vi "To String.vi"(8 "error in (no error)":errorcluster, 11 "Variant in":refnum<class "Variant.lvclass">) -> (0 "error out":errorcluster, 2 "String":string)   [LabVIEW 2020, in "Data.lvlib" / "Variant.lvclass"]
doc: "Convert 'Generic Data in' to a string.\nConvert the variant data to an XML string. The Variant properties will not be extracted."
uses:
  Variant.lvclass
  Variant.lvclass/Variant.ctl
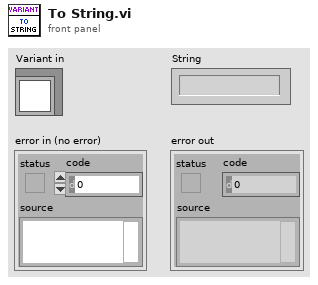
[diagram p1: front panel]
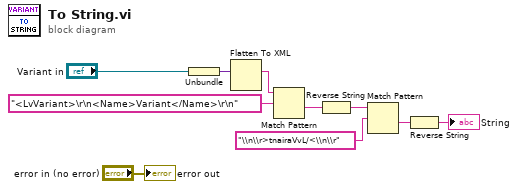
[diagram p0: block diagram]
diagram:
  n1 = Unbundle("Variant in") -> (w8:variant)
  n2 = Flatten To XML(6:w8) -> (2:w6:string)
  n3 = Match Pattern(string=w6, regular expression="<LvVariant>\r\n<Name>Variant</Name>\r\n") -> (after substring=w5:string)  [unwired: 1 in, 3 out]
  n4 = Reverse String(1:w5) -> (0:w4:string)
  n5 = Match Pattern(string=w4, regular expression="\\n\\r>tnairaVvL/<\\n\\r") -> (after substring=w2:string)  [unwired: 1 in, 3 out]
  n6 = Reverse String(1:w2) -> (0:→"String":string)
  "error out" <- "error in (no error)"
